vi "Simon main.vi"() -> ()   [LabVIEW 2020]
uses:
  Simon/State.ctl
  Simon/Application Data.ctl
panel:
  out "The numbe of colors you have memorized!":i32
  out "Keep Entering":bool
  in  "Please enter your answer:":T1
  out "Sequence for Player to Memorize":u32(colorbox)
  # "Simon"
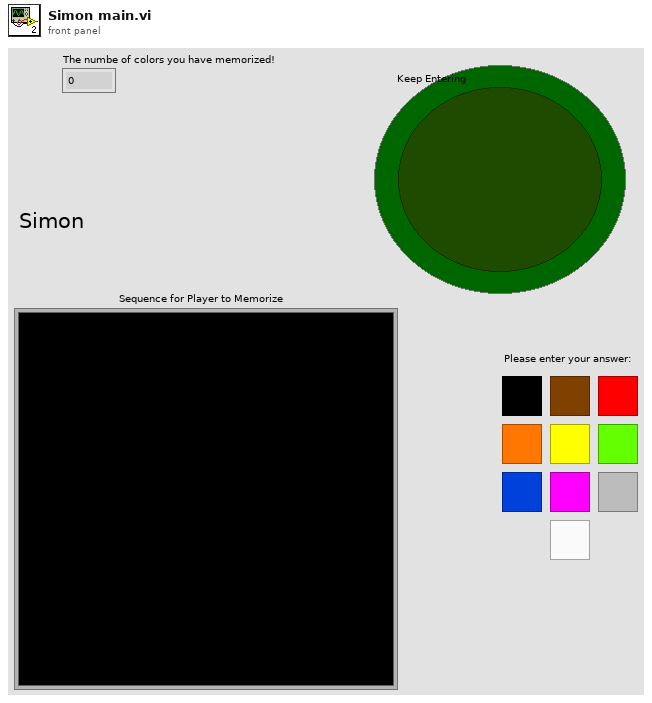
[diagram p1: front panel]
types:
  T1 = cluster{"0":bool, "7":bool, "8":bool, "9":bool, "4":bool, "5":bool, "6":bool, "1":bool, "2":bool, "3":bool}
  T2 = typedef "Application Data.ctl" = cluster{"Sequence ":i32[], "\n Colors":u32[], "Wait Time (ms)":u32, "Last Key":i16, "Nmber of Key Pressed":i32, "Tally":i32, "Keep Entering":bool}
  T3 = typedef "State.ctl" = enum16{"Initialize", "Add New Color", "Show Sequence", "Wait For Event", "Check Key Press", "Success", "Fail", "Exit"}
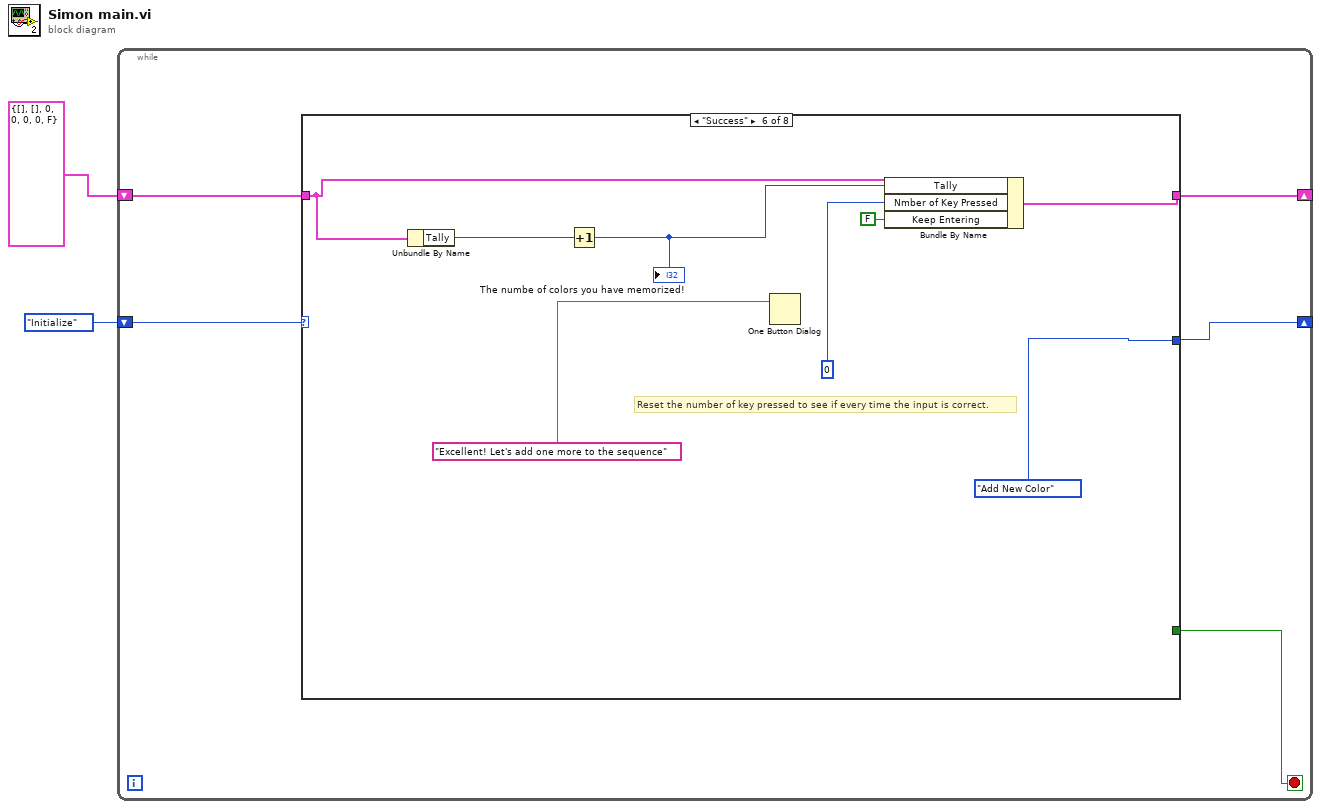
[diagram p0: block diagram]
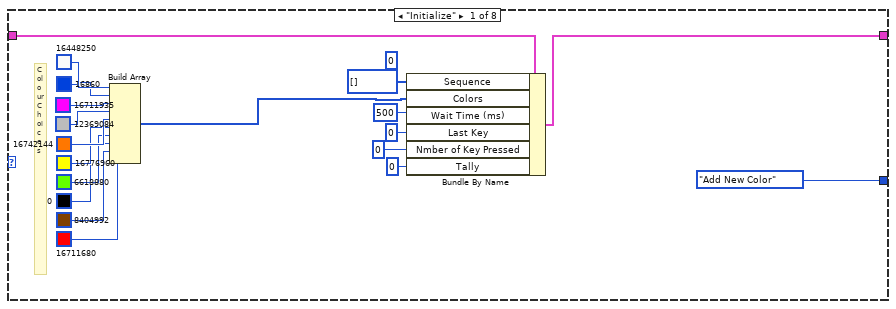
[diagram p2: hidden frame]
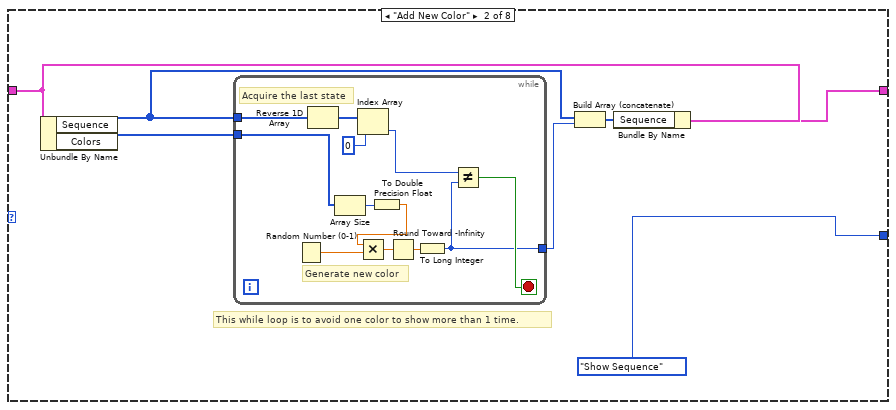
[diagram p3: hidden frame]
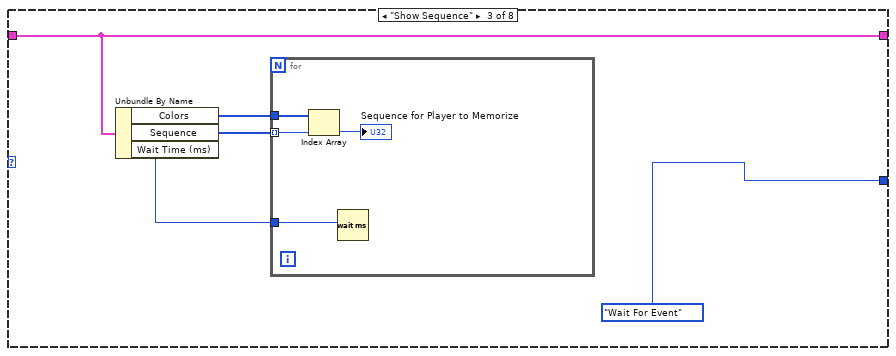
[diagram p4: hidden frame]
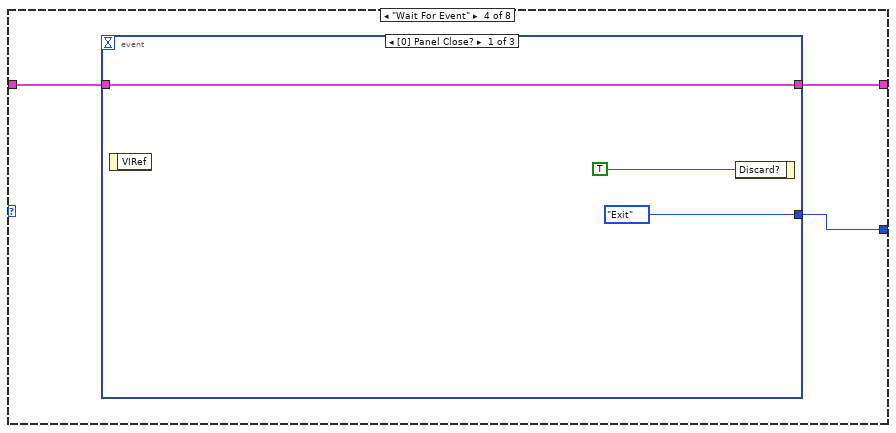
[diagram p5: hidden frame]
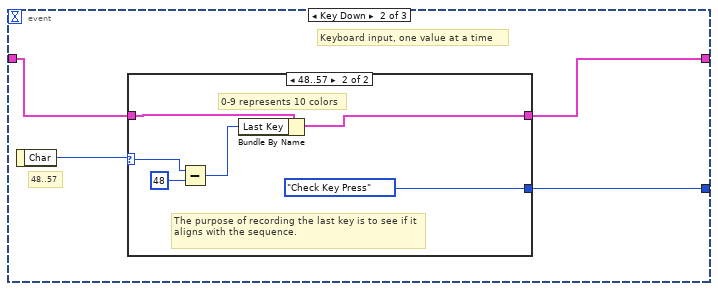
[diagram p6: hidden frame]
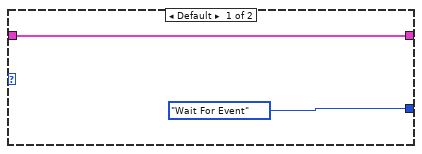
[diagram p7: hidden frame]
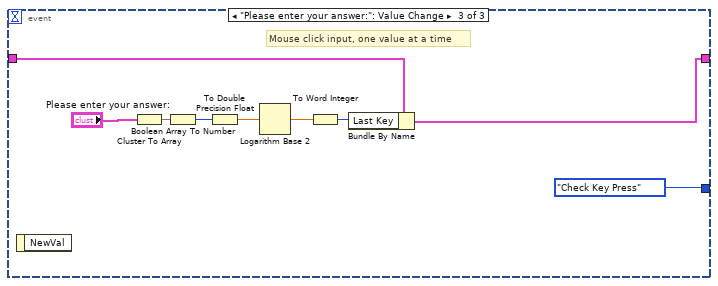
[diagram p8: hidden frame]
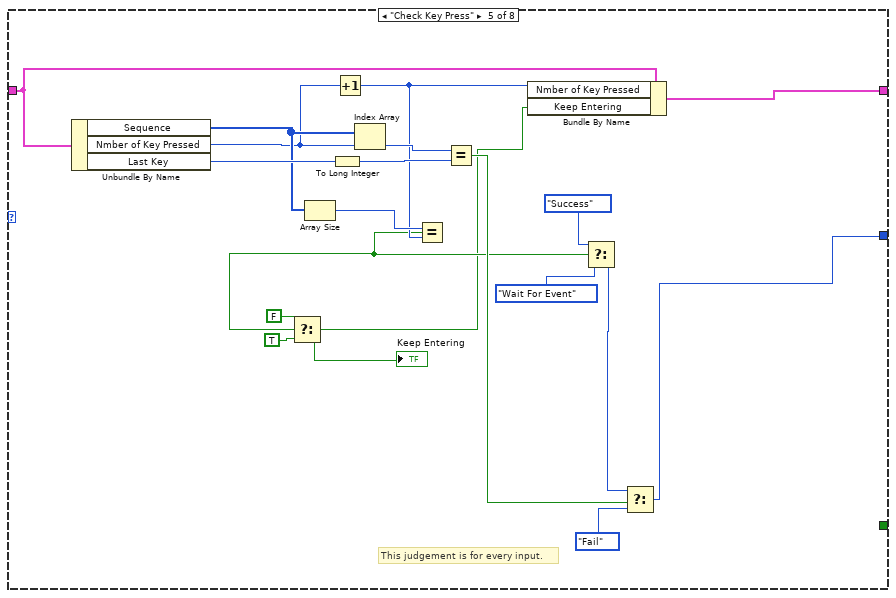
[diagram p9: hidden frame]
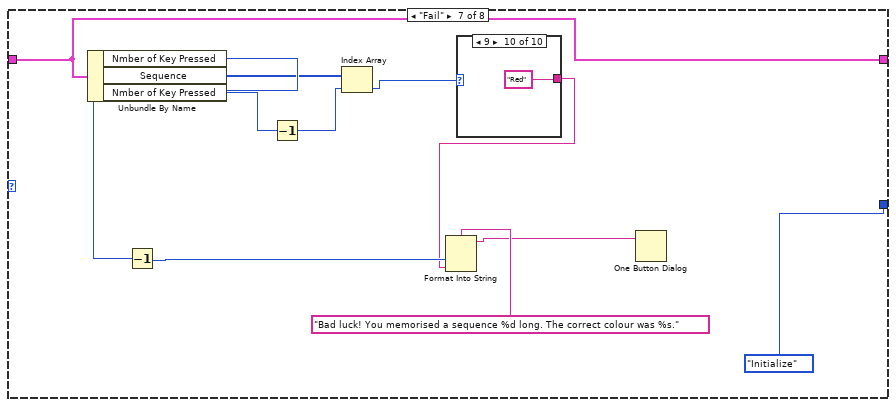
[diagram p10: hidden frame]
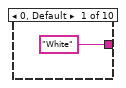
[diagram p11: hidden frame]
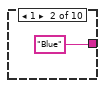
[diagram p12: hidden frame]
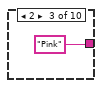
[diagram p13: hidden frame]
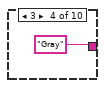
[diagram p14: hidden frame]
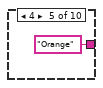
[diagram p15: hidden frame]
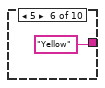
[diagram p16: hidden frame]
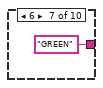
[diagram p17: hidden frame]
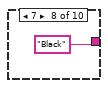
[diagram p18: hidden frame]
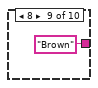
[diagram p19: hidden frame]
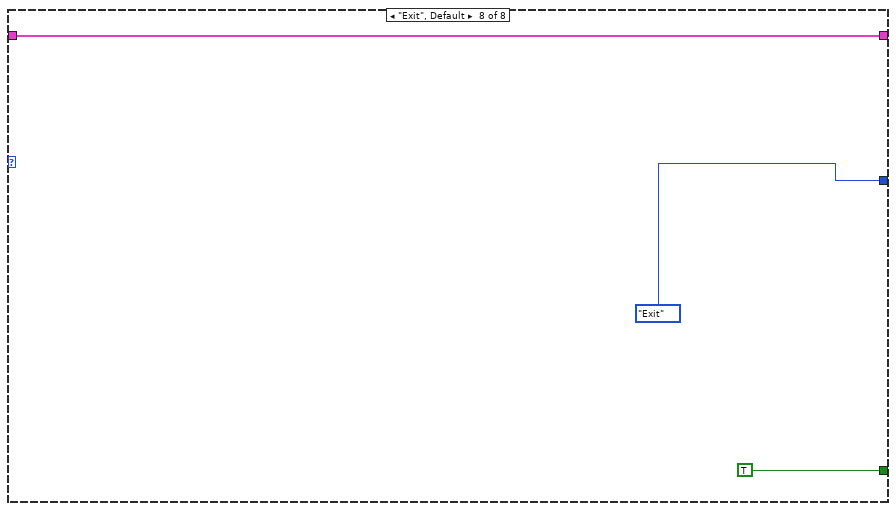
[diagram p20: hidden frame]
diagram:
  n1 = while {
    shift-right: [w4] -> _
    shift-left: T2 {"Sequence "=[], "\n Colors"=[], "Wait Time (ms)"=0, "Last Key"=0, "Nmber of Key Pressed"=0, "Tally"=0, "Keep Entering"=FALSE} -> [w5]
    shift-right: [w3] -> _
    shift-left: State."Initialize" -> [w7]
    stop <- w6 stop-if-true
    n2 = case shown="\"Success\"" w7 {
      tunnel: [_ _ _ _ _ _ _ TRUE] -> w6
      tunnel: w5 -> [w22 w29 w50 w57 w97 w106 w114 w131]
      tunnel: [w21 w28 w50 w56 w96 w105 w114 w131] -> w4
      tunnel: [State."Add New Color" State."Show Sequence" State."Wait For Event" w55 w94 State."Add New Color" State."Initialize" State."Exit"] -> w3
      frame "Initialize" {
        (unwired) 0 ("Wait Time (ms)")
        # "Colour Choices"
        n3 = Build Array(u32 16448250 ("Color Box"), u32 16860 ("Color Box"), u32 16711935 ("Color Box"), u32 12369084 ("Color Box"), u32 16742144 ("Color Box"), u32 16776960 ("Color Box"), u32 6618880 ("Color Box"), u32 0 ("Color Box"), u32 8404992 ("Color Box"), u32 16711680 ("Color Box")) -> (w8:u32[])
        n4 = Bundle By Name(cluster=w22, "Sequence"=i32[] [], "Colors"=w8, "Wait Time (ms)"=u32 500, "Last Key"=i16 0, "Nmber of Key Pressed"=0, "Tally"=0) -> (w21:T2)
      }
      frame "Add New Color" {
        # "This while loop is to avoid one color to show more than 1 time."
        n5 = Unbundle By Name(w29) -> ("Sequence"=w32:i32[], "Colors"=w33:u32[])
        n6 = while {
          tunnel: w32 -> [w45]
          tunnel: w33 -> [w42]
          tunnel: [w34] -> w31
          stop <- w35 stop-if-true
          # "Generate new color"
          # "Acquire the last state"
          n7 = Random Number (0-1)() -> (number: 0 to 1=w41:dbl)
          n8 = Reverse 1D Array(array=w45) -> (reversed array=w44:i32[])
          n9 = Array Size(array=w42) -> (size(s)=w39:i32)
          n10 = Index Array(array=w44, index=0) -> (element=w36:i32)
          n11 = To Double Precision Float(number=w39) -> (double precision float=w38:dbl)
          n12 = Multiply(x=w38, y=w41) -> (x*y=w40:dbl)
          n13 = Round Toward -Infinity(1:w40) -> (0:w37:dbl)
          n14 = To Long Integer(number=w37) -> (32bit integer=w34:i32)
          n15 = Not Equal?(x=w36, y=w34) -> (x != y?=w35:bool)
        }
        n16 = Build Array (concatenate)(w32, w31) -> (w30:i32[])
        n17 = Bundle By Name(cluster=w29, "Sequence"=w30) -> (w28:T2)
      }
      frame "Show Sequence" {
        n18 = Unbundle By Name(w50) -> ("Colors"=w49:u32[], "Sequence"=w48:i32[], "Wait Time (ms)"=w47:u32)
        n19 = for {
          tunnel: w49 -> [w54]
          tunnel: w48 -> [w53] mode=indexing
          tunnel: w47 -> [w51]
          n20 = Index Array(array=w54, index=w53) -> (element=→"Sequence for Player to Memorize":u32)
          n21 = Wait (ms)(milliseconds to wait=w51) -> ()  [unwired: 1 out]
        }
      }
      frame "Wait For Event" {
        n22 = event shown="[0] Panel Close?" {
          selector: _ -> [_ _ _]
          dyn-events: _ -> [_ _ _]
          timeout: _ -> [_ _ _]
          tunnel: w57 -> [w60 w63 w73]
          tunnel: [w60 w62 w74] -> w56
          tunnel: [State."Exit" w61 State."Check Key Press"] -> w55
          event Panel Close? {
            n23 = event-data() -> ()  [unwired: 1 in, 1 out]
            n24 = event-data("Discard?"=TRUE) -> ()  [unwired: 1 in, 1 out]
          }
          event Key Down {
            # "Keyboard input, one value at a time"
            # "48..57"
            n25 = event-data() -> ("Char"=w64:i16)  [unwired: 1 in]
            n26 = case shown="48..57" w64 {
              selector: w64 -> [_ w70]
              tunnel: w63 -> [w66 w72]
              tunnel: [w66 w71] -> w62
              tunnel: [State."Wait For Event" State."Check Key Press"] -> w61
              frame Default {
              }
              frame 48..57 {
                # "The purpose of recording the last key is to see if it aligns with the sequence."
                # "0-9 represents 10 colors"
                n27 = Subtract(x=w70, y=i16 48) -> (x-y=w68:i16)
                n28 = Bundle By Name(cluster=w72, "Last Key"=w68) -> (w71:T2)
              }
            }
          }
          event "Please enter your answer:": Value Change {
            # "Mouse click input, one value at a time"
            n29 = event-data() -> ()  [unwired: 1 in, 1 out]
            n30 = Cluster To Array(cluster="Please enter your answer:") -> (array=w80:bool[])
            n31 = Boolean Array To Number(Boolean array=w80) -> (number=w79:u32)
            n32 = To Double Precision Float(number=w79) -> (double precision float=w78:dbl)
            n33 = Logarithm Base 2(1:w78) -> (0:w77:dbl)
            n34 = To Word Integer(number=w77) -> (16bit integer=w76:i16)
            n35 = Bundle By Name(cluster=w73, "Last Key"=w76) -> (w74:T2)
          }
        }
      }
      frame "Check Key Press" {
        # "This judgement is for every input."
        n36 = Unbundle By Name(w97) -> ("Sequence"=w93:i32[], "Nmber of Key Pressed"=w87:i32, "Last Key"=w98:i16)
        n37 = Array Size(array=w93) -> (size(s)=w92:i32)
        n38 = To Long Integer(number=w98) -> (32bit integer=w99:i32)
        n39 = Increment(x=w87) -> (x+1=w86:i32)
        n40 = Index Array(array=w93, index=w87) -> (element=w100:i32)
        n41 = Equal?(x=w92, y=w86) -> (x = y?=w85:bool)
        n42 = Select(t=FALSE, s=w85, f=TRUE) -> (s? t:f=w82:bool)
        "Keep Entering" <- w82
        n43 = Equal?(x=w100, y=w99) -> (x = y?=w91:bool)
        n44 = Bundle By Name(cluster=w97, "Nmber of Key Pressed"=w86, "Keep Entering"=w82) -> (w96:T2)
        n45 = Select(t=State."Success", s=w85, f=State."Wait For Event") -> (s? t:f=w88:T3)
        n46 = Select(t=w88, s=w91, f=State."Fail") -> (s? t:f=w94:T3)
      }
      frame "Success" {
        # "Reset the number of key pressed to see if every time the input is correct."
        n47 = Unbundle By Name(w106) -> ("Tally"=w108:i32)
        n48 = Increment(x=w108) -> (x+1=w107:i32)
        "The numbe of colors you have memorized!" <- w107
        n49 = One Button Dialog(message="Excellent! Let's add one more to the sequence") -> ()  [unwired: 1 in, 1 out]
        n50 = Bundle By Name(cluster=w106, "Tally"=w107, "Nmber of Key Pressed"=0, "Keep Entering"=FALSE) -> (w105:T2)
      }
      frame "Fail" {
        n51 = Unbundle By Name(w114) -> ("Nmber of Key Pressed"=w118:i32, "Sequence"=w113:i32[], "Nmber of Key Pressed"=w110:i32)
        n52 = Decrement(x=w118) -> (x-1=w117:i32)
        n53 = Decrement(x=w110) -> (x-1=w109:i32)
        n54 = Index Array(array=w113, index=w109) -> (element=w112:i32)
        n55 = case shown="9" w112 {
          tunnel: ["White" "Blue" "Pink" "Gray" "Orange" "Yellow" "GREEN" "Black" "Brown" "Red"] -> w111
          frame 0, Default {
          }
          frame 1 {
          }
          frame 2 {
          }
          frame 3 {
          }
          frame 4 {
          }
          frame 5 {
          }
          frame 6 {
          }
          frame 7 {
          }
          frame 8 {
          }
          frame 9 {
          }
        }
        n56 = Format Into String(format string="Bad luck! You memorised a sequence %d long. The correct colour was %s." ("message"), w117, w111) -> (resulting string=w116:string)  [unwired: 2 in, 1 out]
        n57 = One Button Dialog(message=w116) -> ()  [unwired: 1 in, 1 out]
      }
      frame "Exit", Default {
      }
    }
  }
